vi "02 - Real API list + loop.vi"() -> ()   [LabVIEW 2020]
uses:
  client/client.lvlib
panel:
  out "Array":string[](array[string])
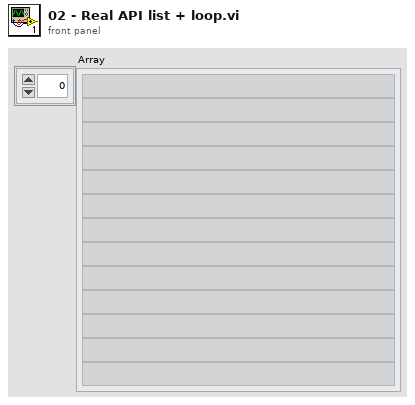
[diagram p1: front panel]
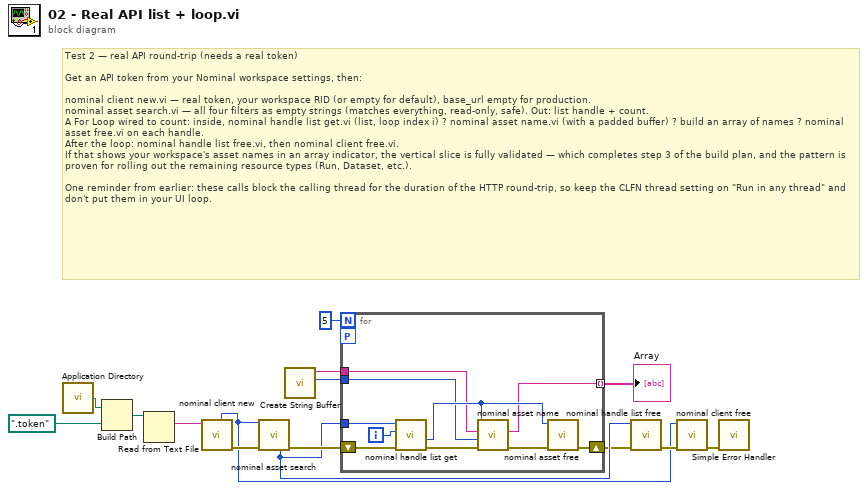
[diagram p0: block diagram]
diagram:
  # "Test 2 — real API round-trip (needs a real token)\n\nGet an API token from your Nominal workspace settings, then:\n\nnominal client new.vi — real token, your workspace RID (or empty for default), base_url empty for production.\nnominal asset search.vi — all four filters as empty strings (matches everything, read-only, safe). Out: list handle + count.\nA For Loop wired to count: inside, nominal handle list get.vi (list, loop index i) ? nominal asset name.vi (with a padded buffer) ? build an array of names ? nominal asset free.vi on each handle.\nAfter the loop: nominal handle list free.vi, then nominal client free.vi.\nIf that shows your workspace's asset names in an array indicator, the vertical slice is fully validated — which completes step 3 of the build plan, and the pattern is proven for rolling out the remaining resource types (Run, Dataset, etc.).\n\nOne reminder from earlier: these calls block the calling thread for the duration of the HTTP round-trip, so keep the CLFN thread setting on \"Run in any thread\" and don't put them in your UI loop."
  n1 = call <vilib>:"Application Directory.vi"() -> ("Application Directory"=w7:path)
  n2 = Build Path(base path=w7, name or relative path=path ".token") -> (appended path=w5:path)
  n3 = Read from Text File(file (use dialog)=w5) -> (text=w4:string)  [unwired: 3 in, 3 out]
  n4 = call "nominal client new.vi"("token"=w4) -> ("error out"=w14:errorcluster, "out_client out"=w10:i32)  [unwired: 8 in, 1 out]
  n5 = call "nominal asset search.vi"("client"=w10, "error in (no error)"=w14) -> ("out_list out"=w13:i32, "error out"=w15:errorcluster)  [unwired: 10 in, 2 out]
  n6 = call "Create String Buffer.vi"() -> ("dub Buffer Size"=w1:i32, "String Buffer"=w2:string)  [unwired: 9 in, 1 out]
  n7 = for {
    N: 5 -> [_]
    tunnel: w13 -> [w25]
    shift-right: [w19] -> w12
    shift-left: w15 -> [w20]
    tunnel: w2 -> [w18]
    tunnel: w1 -> [w17]
    tunnel: [w16] -> w8 mode=indexing
    workers-P: _ -> [_]
    i -> [w23]
    n8 = call "nominal handle list get.vi"("error in (no error)"=w20, "index"=w23, "list"=w25) -> ("error out"=w21:errorcluster, "out_handle out"=w24:i32)  [unwired: 6 in, 1 out]
    n9 = call "nominal asset name.vi"("error in (no error)"=w21, "cap"=w17, "buf"=w18, "asset"=w24) -> ("error out"=w22:errorcluster, "buf out"=w16:string)  [unwired: 4 in, 2 out]
    n10 = call "nominal asset free.vi"("error in (no error)"=w22, "asset"=w24) -> ("error out"=w19:errorcluster)  [unwired: 8 in, 1 out]
  }
  "Array" <- w8
  n11 = call "nominal handle list free.vi"("error in (no error)"=w12, "list"=w13) -> ("error out"=w11:errorcluster)  [unwired: 8 in, 1 out]
  n12 = call "nominal client free.vi"("error in (no error)"=w11, "client"=w10) -> ("error out"=w9:errorcluster)  [unwired: 8 in, 1 out]
  n13 = call <vilib>:"Simple Error Handler.vi"("error in (no error)"=w9) -> ()  [unwired: 4 in, 5 out]
